vi "Write MSG Center.vi"(8 "error in (no error)":errorcluster, 10 "MSG Center":refnum<vi>, 11 "Domino Laser module Class in":refnum<class "Domino Laser module Class.lvclass">) -> (0 "error out":errorcluster, 3 "Domino Laser module Class out":refnum<class "Domino Laser module Class.lvclass">)   [LabVIEW 2015, in "Domino LM.lvlib" / "Domino Laser module Class.lvclass"]
uses:
  CTRLS/Domino Laser module Class.lvclass
  CTRLS/Domino Laser module Class.lvclass/Domino Laser module Class.ctl
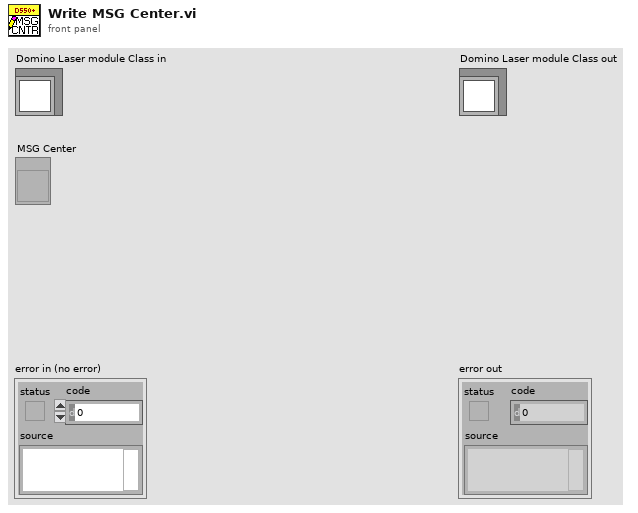
[diagram p1: front panel]
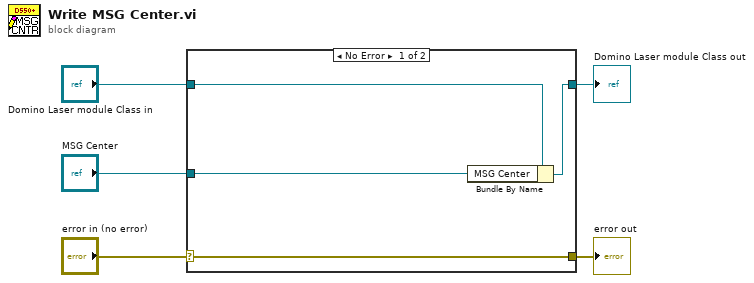
[diagram p0: block diagram]
diagram:
  n1 = case shown="No Error" "error in (no error)" {
    selector: "error in (no error)" -> [w9 w10]
    tunnel: [w9 w10] -> w4
    tunnel: [w7 w11] -> w2
    tunnel: "Domino Laser module Class in" -> [w8 w11]
    tunnel: "MSG Center" -> [w6 _]
    frame No Error {
      n2 = Bundle By Name(cluster=w8, "MSG Center"=w6) -> (w7:refnum<class "Domino Laser module Class.lvclass">)
    }
    frame Error {
    }
  }
  "error out" <- w4
  "Domino Laser module Class out" <- w2
